vi "BRig_dataLC_ENL2_First_Count_l2.vi"() -> (2 "output_ENL2_First_Count_l2":i32)   [LabVIEW 2014]
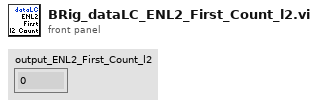
[diagram p1: front panel]
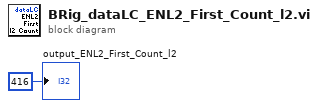
[diagram p0: block diagram]
diagram:
  "output_ENL2_First_Count_l2" <- 416 ("output_iBlock")
